vi "Error Query.vi"(0 "VISA resource name":refnum<visa-resource-name>, 11 "error in (no error)":errorcluster) -> (4 "VISA resource name out":refnum<visa-resource-name>, 8 "Error":i32, 10 "Error Message":string, 15 "error out":errorcluster)   [LabVIEW 2020, in "Keithley 27XX.lvlib"]
doc: "This VI reads an error code and a message from the instrument's error queue.\n\nNote:\nThis VI is called automatically by most driver VIs so it is not usually necessary to call this in an application."
uses:
  Keithley 27XX.lvlib
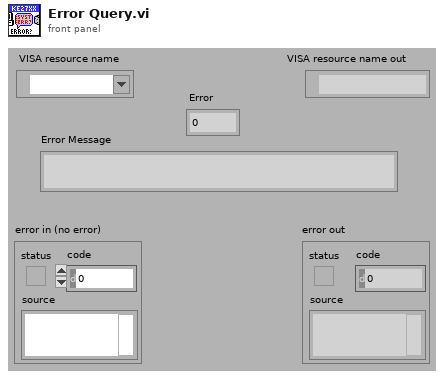
[diagram p1: front panel]
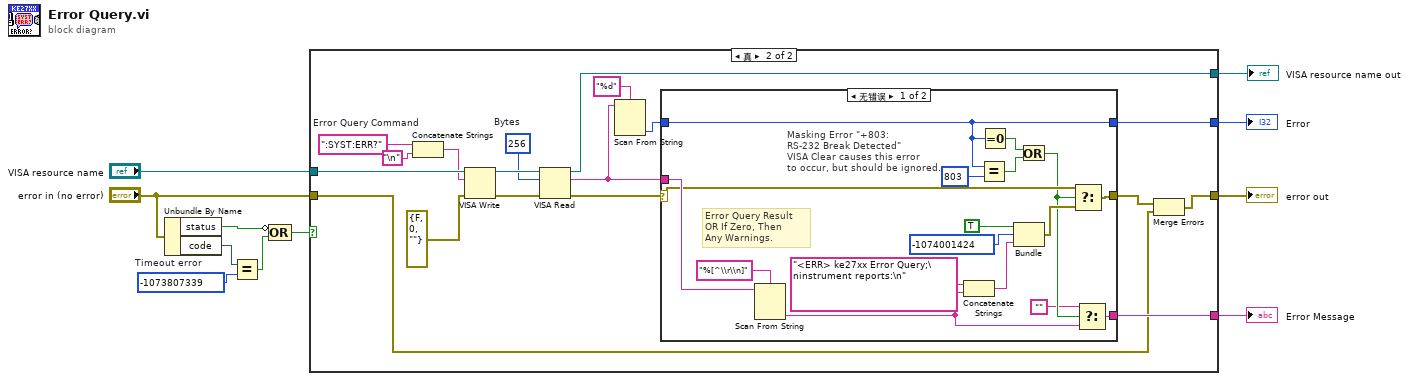
[diagram p0: block diagram]
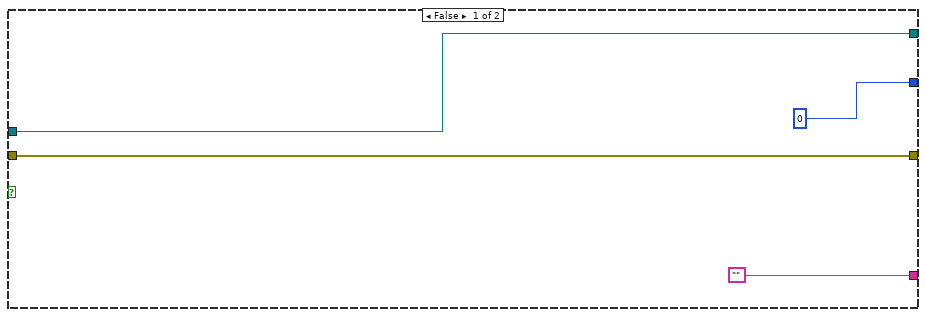
[diagram p2: hidden frame]
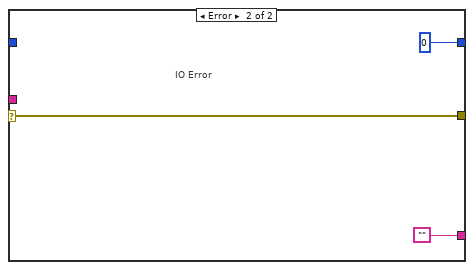
[diagram p3: hidden frame]
diagram:
  w4 = -1073807339  # Timeout error
  n1 = Unbundle By Name("error in (no error)") -> ("status"=w5:bool, "code"=w2:i32)
  n2 = Equal?(x=w2, y=w4) -> (x = y?=w3:bool)
  n3 = Compound Arithmetic op=OR(invert w5, w3) -> (w1:bool)
  n4 = case shown="真" w1 {
    tunnel: ["" w33] -> w11
    tunnel: [0 w32] -> w10
    tunnel: [w15 w31] -> w9
    tunnel: "VISA resource name" -> [w15 w30]
    tunnel: "error in (no error)" -> [w12 w24]
    tunnel: [w12 w23] -> w7
    frame False {
    }
    frame True {
      w28 = u32 256  # Bytes
      w17 = ":SYST:ERR?"  # Error Query Command
      n5 = Concatenate Strings(w17, "\n") -> (w16:string)
      n6 = VISA Write(VISA resource name=w30, write buffer=w16, error in (no error)=errorcluster {"status"=FALSE, "code"=0, "source"=""}) -> (VISA resource name out=w29:refnum<visa-resource-name>, error out=w27:errorcluster)  [unwired: 1 out]
      n7 = VISA Read(VISA resource name=w29, byte count=w28, error in (no error)=w27) -> (VISA resource name out=w31:refnum<visa-resource-name>, read buffer=w22:string, error out=w19:errorcluster)  [unwired: 1 out]
      n8 = Scan From String(format string="%d", input string=w22) -> (output 1=w20:i32)  [unwired: 3 in, 3 out]
      n9 = case shown="无错误" w19 {
        selector: w19 -> [w42 w51]
        tunnel: w22 -> [w43 _]
        tunnel: [w46 w51] -> w25
        tunnel: [w37 ""] -> w33
        tunnel: [w40 0] -> w32
        tunnel: w20 -> [w40 _]
        frame No Error {
          # "Masking Error \"+803:\nRS-232 Break Detected\"\nVISA Clear causes this error\nto occur, but should be ignored."
          # "Error Query Result\nOR If Zero, Then\nAny Warnings."
          n10 = Scan From String(format string="%[^\\r\\n]", input string=w43) -> (output 1=w35:string)  [unwired: 3 in, 3 out]
          n11 = Concatenate Strings("<ERR> ke27xx Error Query;\ninstrument reports:\n" ("Source"), w35) -> (w48:string)
          n12 = Equal?(x=w40, y=803) -> (x = y?=w38:bool)
          n13 = Equal To 0?(x=w40) -> (x = 0?=w39:bool)
          n14 = Bundle("Status"=TRUE, "Code"=-1074001424, w48) -> (w47:cluster{"Status":bool, "Code":i32, string})  [unwired: 1 in]
          n15 = Or(x=w39, y=w38) -> (x .or. y?=w36:bool)
          n16 = Select(t=w42, s=w36, f=w47) -> (s? t:f=w46:errorcluster)
          n17 = Select(t="", s=w36, f=w35) -> (s? t:f=w37:string)
        }
        frame Error {
          # "IO Error"
        }
      }
      n18 = Merge Errors(w25, w24) -> (w23:errorcluster)
    }
  }
  "Error Message" <- w11
  "Error" <- w10
  "VISA resource name out" <- w9
  "error out" <- w7
